vi "Execute Utility.vi"(0 "resource":string, 1 "verbose?":bool, 5 "bitfile":path, 7 "serdes":string, 9 "script":path, 11 "error in":errorcluster) -> (4 "standard output":string, 6 "standard error":string, 8 "return code":i32, 15 "error out":errorcluster)   [LabVIEW 2025, in "I2C Bus Monitor.lvclass"]
uses:
  <vilib>/regexp/Match Regular Expression.xnode
  I2C Bus Monitor.lvclass
  I2C Bus Monitor.lvclass/I2C Bus Monitor.ctl
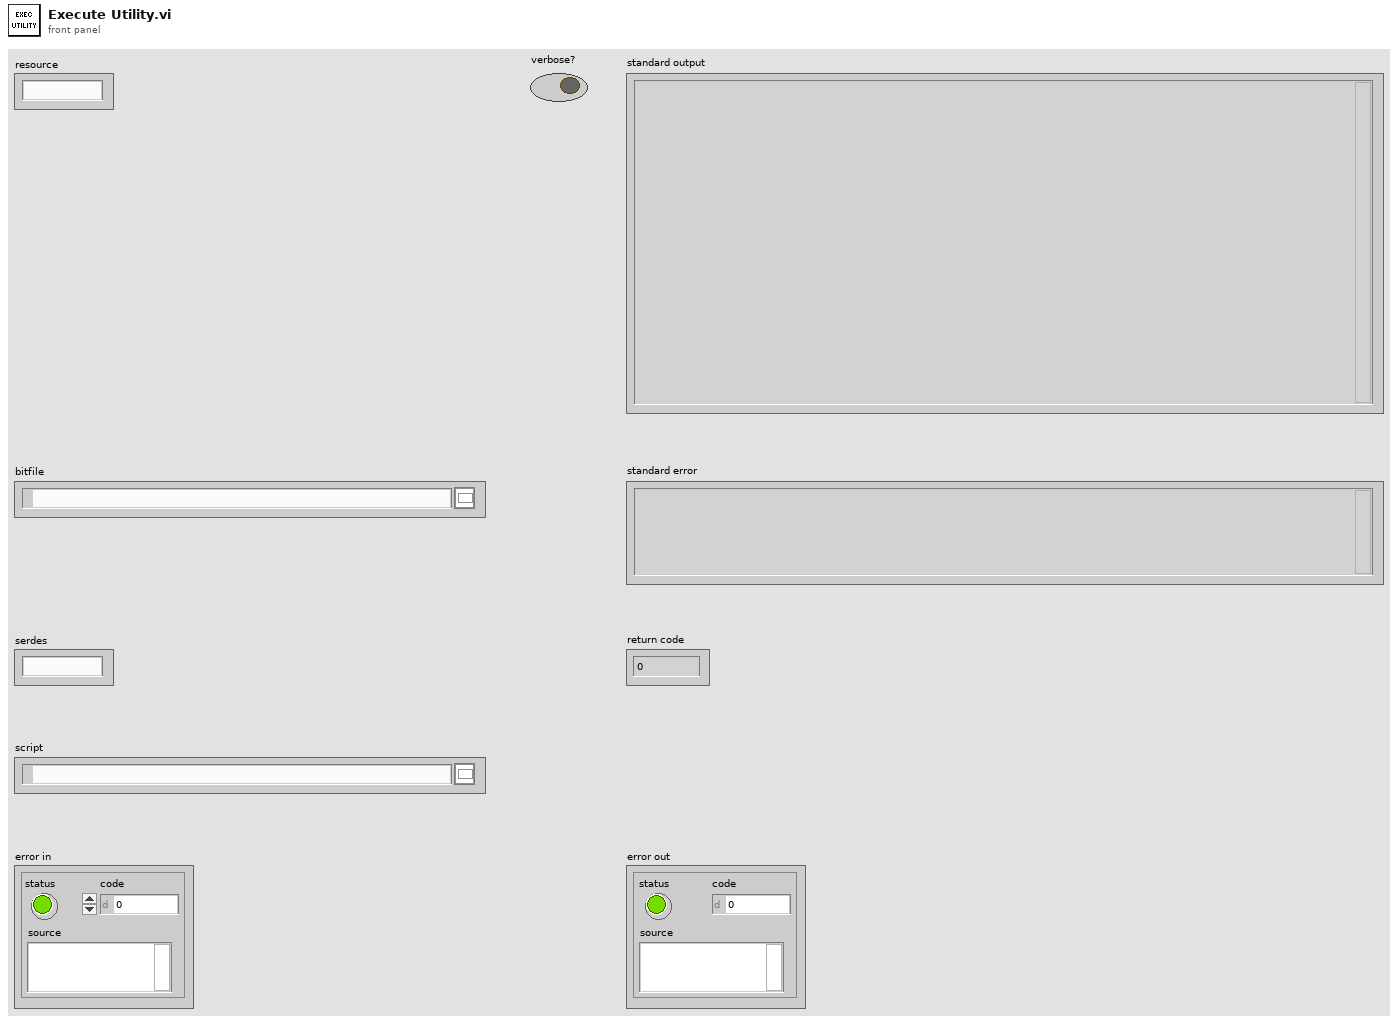
[diagram p1: front panel]
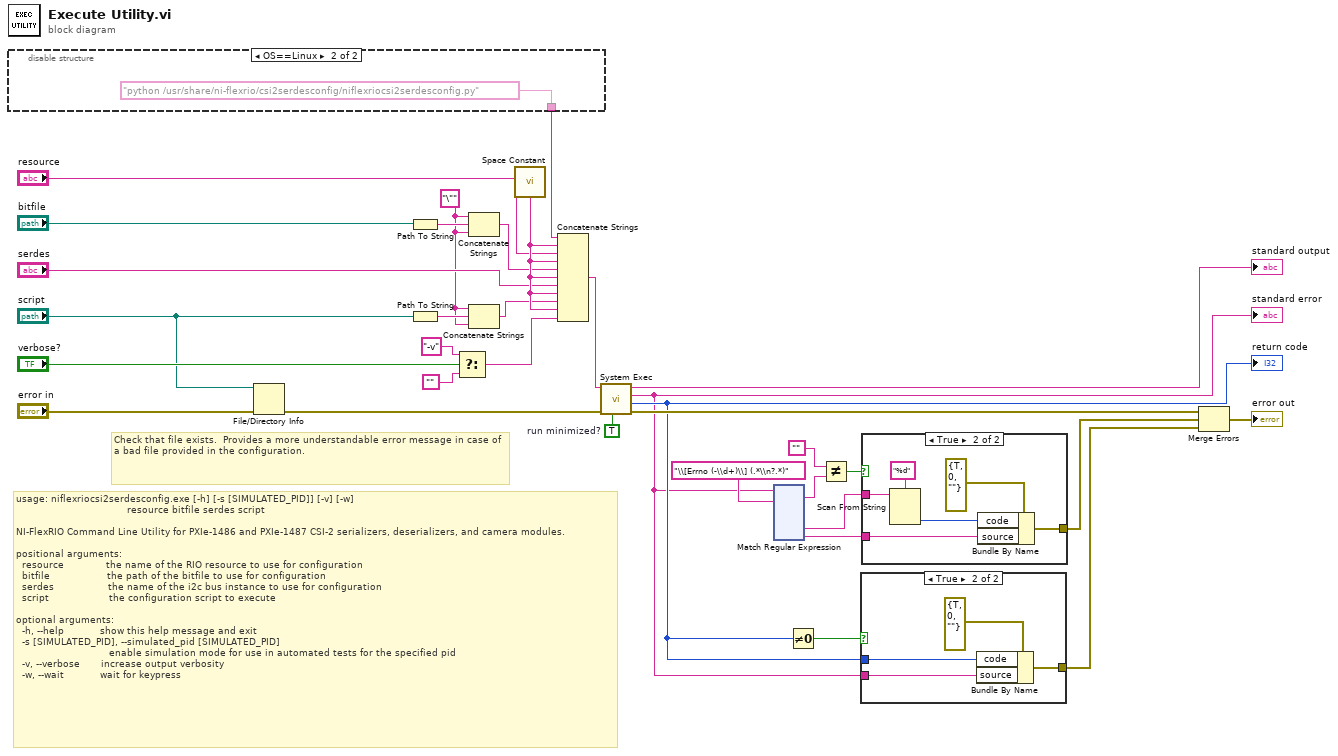
[diagram p0: block diagram]
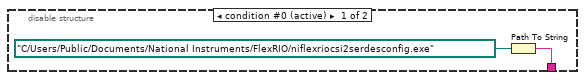
[diagram p3: hidden frame]
diagram:
  w11 = TRUE  # run minimized?
  w21 = "\""
  # "Check that file exists.  Provides a more understandable error message in case of a bad file provided in the configuration."
  # "usage: niflexriocsi2serdesconfig.exe [-h] [-s [SIMULATED_PID]] [-v] [-w]\n                                     resource bitfile serdes script\n\nNI-FlexRIO Command Line Utility for PXIe-1486 and PXIe-1487 CSI-2 serializers, deserializers, and camera modules.\n\npositional arguments:\n  resource              the name of the RIO resource to use for configuration\n  bitfile                   the path of the bitfile to use for configuration\n  serdes                  the name of the i2c bus instance to use for configuration\n  script                    the configuration script to execute\n\noptional arguments:\n  -h, --help            show this help message and exit\n  -s [SIMULATED_PID], --simulated_pid [SIMULATED_PID]\n                               enable simulation mode for use in automated tests for the specified pid\n  -v, --verbose       increase output verbosity\n  -w, --wait            wait for keypress"
  n1 = disable-structure shown="OS==Linux" {
    disable-tunnel: [w35 "python /usr/share/ni-flexrio/csi2serdesconfig/niflexriocsi2serdesconfig.py"] -> w10
    frame condition #0 (active) {
      n2 = Path To String(path=path "C:/Users/Public/Documents/National Instruments/FlexRIO/niflexriocsi2serdesconfig.exe") -> (string=w35:string)
    }
    frame condition #1 {
    }
  }
  n3 = File/Directory Info(path="script", error in="error in") -> (error out=w8:errorcluster)  [unwired: 6 out]
  n4 = Path To String(path="bitfile") -> (string=w22:string)
  n5 = Path To String(path="script") -> (string=w31:string)
  n6 = Select(t="-v", s="verbose?", f="") -> (s? t:f=w16:string)
  n7 = Concatenate Strings(w21, w22, w21) -> (w23:string)
  n8 = Concatenate Strings(w21, w31, w21) -> (w32:string)
  n9 = call <vilib>:"Space Constant.vi"() -> ("String"=w33:string)
  n10 = Concatenate Strings(w10, w33, "resource", w33, w23, w33, "serdes", w33, w32, w33, w16) -> (w24:string)
  n11 = call <vilib>:"System Exec.vi"("run minimized? (F)"=w11, "error in (no error)"=w8, "command line"=w24) -> ("error out"=w6:errorcluster, "return code"=w4:i32, "standard error"=w3:string, "standard output"=→"standard output":string)  [unwired: 5 in]
  "standard error" <- w3
  "return code" <- w4
  n12 = xnode "Match Regular Expression"("input string"=w3, "regular expression"="\\[Errno (-\\d+)\\] (.*\\n?.*)") -> ("whole match"=w25:string, "submatch 1"=w13:string, "submatch 2"=w12:string)  [unwired: 4 in, 4 out]
  n13 = Not Equal To 0?(x=w4) -> (x != 0?=w5:bool)
  n14 = Not Equal?(x="", y=w25) -> (x != y?=w26:bool)
  n15 = case shown="True" w5 {
    tunnel: [_ w38] -> w1
    tunnel: w3 -> [_ w39]
    tunnel: w4 -> [_ w37]
    frame False {
    }
    frame True {
      n16 = Bundle By Name(cluster=errorcluster {"status"=TRUE, "code"=0, "source"=""} ("error out"), "code"=w37, "source"=w39) -> (w38:errorcluster)
    }
  }
  n17 = case shown="True" w26 {
    tunnel: [_ w41] -> w2
    tunnel: w13 -> [_ w45]
    tunnel: w12 -> [_ w42]
    frame False {
    }
    frame True {
      n18 = Scan From String(format string="%d", input string=w45) -> (output 1=w43:i32)  [unwired: 3 in, 3 out]
      n19 = Bundle By Name(cluster=errorcluster {"status"=TRUE, "code"=0, "source"=""} ("error out"), "code"=w43, "source"=w42) -> (w41:errorcluster)
    }
  }
  n20 = Merge Errors(w6, w2, w1) -> (→"error out":errorcluster)
